vi "GFITS_Write2DHdrs.vi"(6 "mext":bool, 7 "extension":i32, 8 "error in (no error)":errorcluster, 10 "keys":string[][](array[string]), 11 "fref":u64) -> (0 "error out":errorcluster)   [LabVIEW 2016]
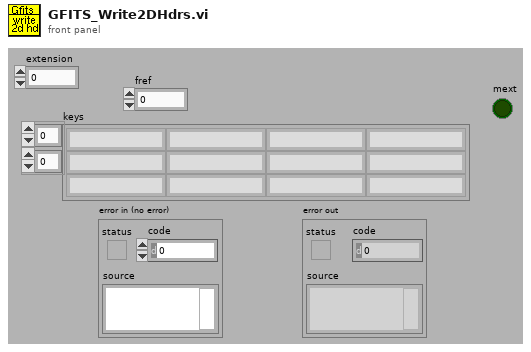
[diagram p1: front panel]
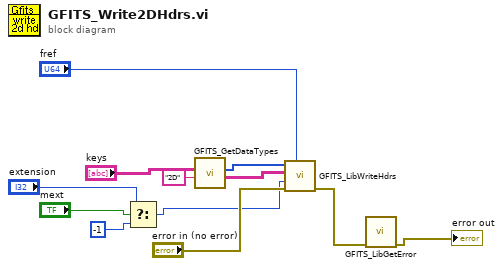
[diagram p0: block diagram]
diagram:
  n1 = Select(t="extension", s="mext", f=-1 ("dnum")) -> (s? t:f=w2:i32)
  n2 = call "GFITS_GetDataTypes.vi"("type"="2D", "keys"="keys") -> ("keys out"=w9:string[][], "datatypes"=w8:i32[])  [unwired: 8 out]
  n3 = call "GFITS_LibWriteHdrs.vi"("file ref"="fref", "error in (no error)"="error in (no error)", "dnum"=w2, "Table In"=w9, "data type"=w8) -> ("error out"=w6:errorcluster)  [unwired: 6 out]
  n4 = call "GFITS_LibGetError.vi"("error in (no error)"=w6) -> ("error out"=→"error out":errorcluster)  [unwired: 10 out]
